vi "Initialize FPGA Resource.vi"(8 "Error In":errorcluster, 10 "FPGA VI Reference":T1, 11 "Display In":refnum<class "Display.lvclass">) -> (0 "Error Out":errorcluster, 3 "Display Out":refnum<class "Display.lvclass">)   [LabVIEW 2019, in "Display.lvclass"]
uses:
  Display.lvclass
  Controls/FPGA Reference.ctl
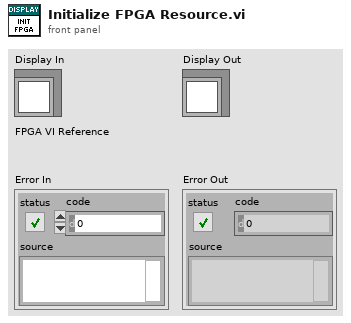
[diagram p1: front panel]
types:
  T1 = typedef "Display.lvclass/FPGA Reference.ctl" = refnum<k20>
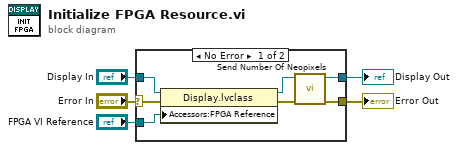
[diagram p0: block diagram]
diagram:
  n1 = case shown="No Error" "Error In" {
    selector: "Error In" -> [w9 w13]
    tunnel: "Display In" -> [w8 w14]
    tunnel: [w11 w14] -> w3
    tunnel: [w10 w13] -> w2
    tunnel: "FPGA VI Reference" -> [w12 _]
    frame No Error {
      n2 = property class="Display.lvclass"(reference=w8, error in=w9, "Accessors:FPGA Reference"=w12) -> (reference out=w6:refnum<class "Display.lvclass">, error out=w7:errorcluster)
      n3 = call "Send Number Of Neopixels.vi"("Error In"=w7, "Display In"=w6) -> ("Error Out"=w10:errorcluster, "Display Out"=w11:refnum<class "Display.lvclass">)  [unwired: 8 in]
    }
    frame Error {
    }
  }
  "Display Out" <- w3
  "Error Out" <- w2
